vi "Processing Step.vi"(8 "error in (no error)":errorcluster, 11 "Handler in":refnum<class "Handler.lvclass">) -> (0 "error out":errorcluster, 2 "Array":T1[](array[typedef]), 3 "Handler out":refnum<class "Handler.lvclass">)   [LabVIEW 2020, in "HTTP Server.lvlib" / "Handler.lvclass"]
doc: "Specifies the step(s) that a handler will be run at as an array to allow a single handler that can be used at multiple steps. To run during multiple steps the handler must inherit from all the desired handler type interfaces and this Processing Step.vi can be manually overridden to specify all the desired steps."
uses:
  Handler.lvclass
  Processing Step.ctl
  HTTP Server.lvlib
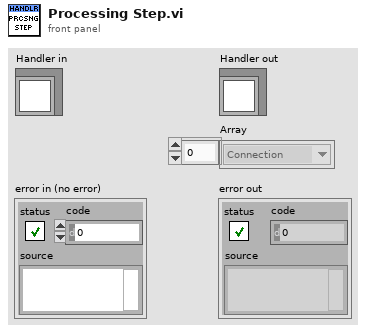
[diagram p1: front panel]
types:
  T1 = typedef "HTTP Server.lvlib/Processing Step.ctl" = enum16{"Connection", "Request", "Routing", "Controller Init", "Controller", "Response", "Complete", "Exception"}
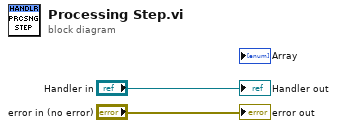
[diagram p0: block diagram]
diagram:
  "error out" <- "error in (no error)"
  "Handler out" <- "Handler in"
